vi "Display Documentation.vi"   [LabVIEW 2025]
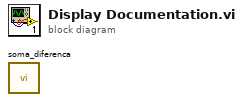
[diagram p0: block diagram]
diagram:
  n1 = call "soma_diferenca.vi"() -> ()  [unwired: 10 in, 2 out]
